vi "[GV]_Lidar 필터 최대거리 (mm).vi"() -> ()   [LabVIEW 2016]
panel:
  in  "Lidar 필터 최대거리 (mm)":dbl=25000.0
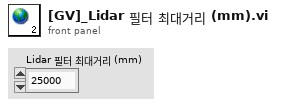
[diagram p1: front panel]
diagram:
